vi "_Remote Send Turbo Command.vi"(4 "error in (no error)":errorcluster, 6 "Input Value":i32, 7 "Pump Command":T1) -> (0 "error out":errorcluster, 1 "Data":string, 2 "Raw Reply":string, 3 "Telegram":string)   [LabVIEW 2012]
uses:
  Type/_Pump Parameter.ctl
  Type/_RT Command.ctl
  Type/_RT Serial Command.ctl
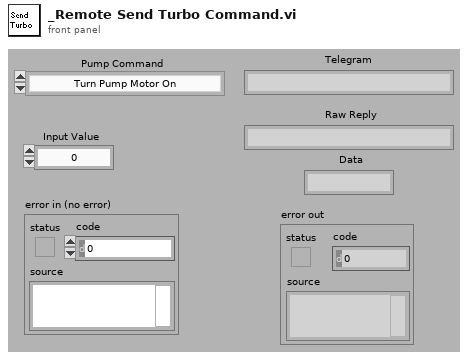
[diagram p1: front panel]
types:
  T1 = typedef "_Pump Parameter.ctl" = enum16{"Turn Pump Motor On", "Turn Pump Motor Off", "Read Pump Oil Deficiency", "Read Rotation Switch Point Attained", "Read Ele. Drive Over Temperature", "Read Pump Over Temperature", "Read Set Rotation Speed Attained", "Read Turbopump Accelerates", "Read Actual Rotation Speed in Hz", "Read Motor Current in A", "Read Operating Hours in h", "Read Motor Voltage in V", "Read Motor Power in W", "Set Rotation Speed Switchpoint in %", "Clear Error", "Read Error Code", "Read Bearing Temperature", "Read Hardware Version", "Read Firmware Version", "Read Operating Hours (Drive)", "Read Rotational Speed (rpm)", "Read Power Stage Temperature", "Read Electronics Temperature", "Read Upper Pump Temperature", "Read Motor Temperature", "Read Error Code History, 1", "Read Error Code History, 2", "Read Error Code History, 3", "Read Error Code History, 4", "Read Error Code History, 5", "Read Error Code History, 6", "Read Error Code History, 7", "Read Error Code History, 8", "Read Error Code History, 9", "Read Error Code History, 10"}
  T2 = typedef "_RT Serial Command.ctl" = cluster{"Port Type":u16, "baud rate (9600)":u32, "data bits (8)":u16, "stop bits (1)":u16, "parity (0:none)":u16, "DoRead":bool, "Command":string}
  T3 = typedef "_RT Command.ctl" = enum16{"Start", "Stop", "Runtime Update", "Get Data", "Get Info", "Get Status", "Get Param", "Get Config", "Get Table", "Read ADC", "Set Oscillator", "Update Config", "Update Table", "Set All Pol", "Set Pol and DC", "Set Max Mass", "Toggle RP", "Toggle EL", "Set PIC", "Initialize Turbo", "Send Turbo Comm", "Close Turbo", "P1", "P2", "P3", "Send Serial", "Set LC Out", "Get LC In", "Read VAC", "Test Table", "Toggle Power", "Get Startup", "Set Startup", "Get ADC Table", "Set ADC Table", "Get Brief Status", "Get Detail Status", "Auxiliary Update", "Set CC Logics", "Set CC Input Logics", "Ignore Error"}
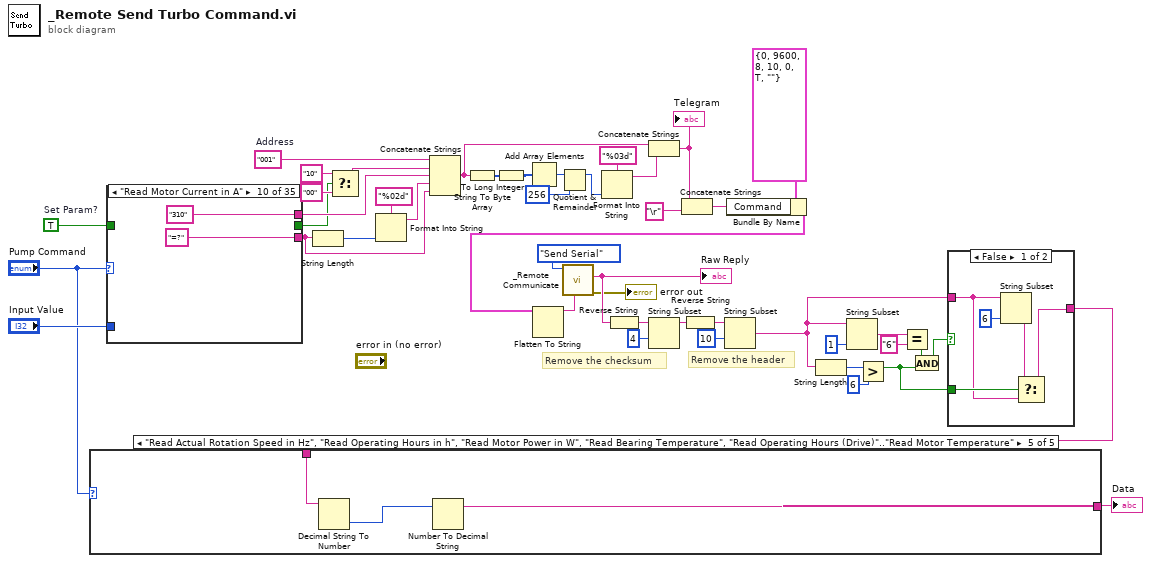
[diagram p0: block diagram]
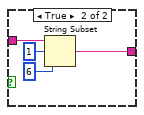
[diagram p2: hidden frame]
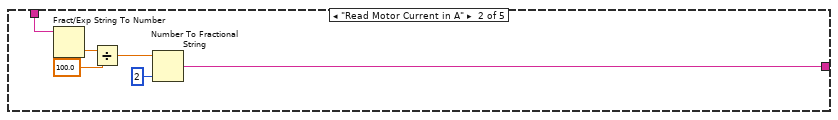
[diagram p4: hidden frame]
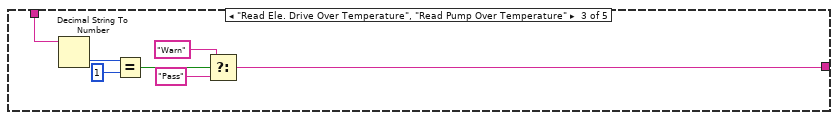
[diagram p5: hidden frame]
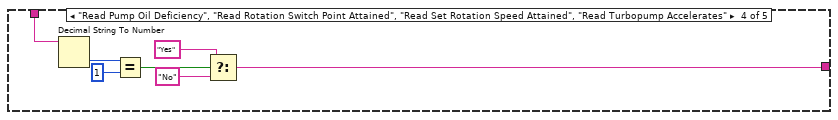
[diagram p6: hidden frame]
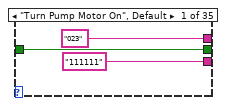
[diagram p7: hidden frame]
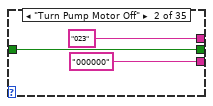
[diagram p8: hidden frame]
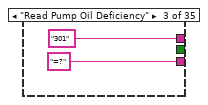
[diagram p9: hidden frame]
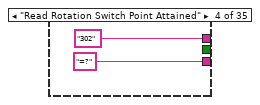
[diagram p10: hidden frame]
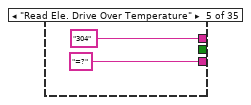
[diagram p11: hidden frame]
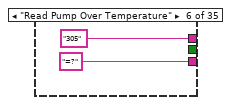
[diagram p12: hidden frame]
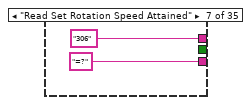
[diagram p13: hidden frame]
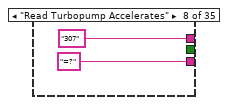
[diagram p14: hidden frame]
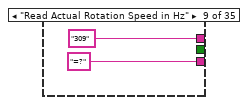
[diagram p15: hidden frame]
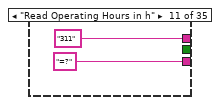
[diagram p16: hidden frame]
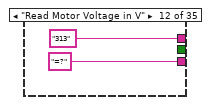
[diagram p17: hidden frame]
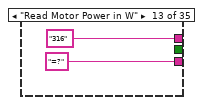
[diagram p18: hidden frame]
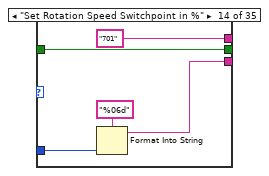
[diagram p19: hidden frame]
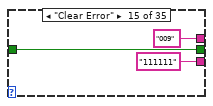
[diagram p20: hidden frame]
diagram:
  w40 = "001"  # Address
  w44 = TRUE  # Set Param?
  # "Remove the header"
  # "Remove the checksum"
  n1 = case shown="\"Read Motor Current in A\"" "Pump Command" {
    tunnel: w44 -> [w49 w50 _ _ _ _ _ _ _ _ _ _ _ w78 w81 _ _ _ _ _ _ _ _ _ _ _ _ _ _ _ _ _ _ _ _]
    tunnel: [w49 w50 _ _ _ _ _ _ _ _ _ _ _ w78 w81 _ _ _ _ _ _ _ _ _ _ _ _ _ _ _ _ _ _ _ _] -> w34
    tunnel: ["023" "023" "301" "302" "304" "305" "306" "307" "309" "310" "311" "313" "316" "701" "009" "303" "342" "354" "312" "314" "398" "324" "326" "330" "346" "360" "361" "362" "363" "364" "365" "366" "367" "368" "369"] -> w35
    tunnel: ["111111" "000000" "=?" "=?" "=?" "=?" "=?" "=?" "=?" "=?" "=?" "=?" "=?" w75 "111111" "=?" "=?" "=?" "=?" "=?" "=?" "=?" "=?" "=?" "=?" "=?" "=?" "=?" "=?" "=?" "=?" "=?" "=?" "=?" "=?"] -> w33
    tunnel: "Input Value" -> [_ _ _ _ _ _ _ _ _ _ _ _ _ w77 _ _ _ _ _ _ _ _ _ _ _ _ _ _ _ _ _ _ _ _ _]
    frame "Turn Pump Motor On", Default {
    }
    frame "Turn Pump Motor Off" {
    }
    frame "Read Pump Oil Deficiency" {
    }
    frame "Read Rotation Switch Point Attained" {
    }
    frame "Read Ele. Drive Over Temperature" {
    }
    frame "Read Pump Over Temperature" {
    }
    frame "Read Set Rotation Speed Attained" {
    }
    frame "Read Turbopump Accelerates" {
    }
    frame "Read Actual Rotation Speed in Hz" {
    }
    frame "Read Motor Current in A" {
    }
    frame "Read Operating Hours in h" {
    }
    frame "Read Motor Voltage in V" {
    }
    frame "Read Motor Power in W" {
    }
    frame "Set Rotation Speed Switchpoint in %" {
      n2 = Format Into String(format string="%06d", w77) -> (resulting string=w75:string)  [unwired: 2 in, 1 out]
    }
    frame "Clear Error" {
    }
    frame "Read Error Code" {
    }
    frame "Read Bearing Temperature" {
    }
    frame "Read Hardware Version" {
    }
    frame "Read Firmware Version" {
    }
    frame "Read Operating Hours (Drive)" {
    }
    frame "Read Rotational Speed (rpm)" {
    }
    frame "Read Power Stage Temperature" {
    }
    frame "Read Electronics Temperature" {
    }
    frame "Read Upper Pump Temperature" {
    }
    frame "Read Motor Temperature" {
    }
    frame "Read Error Code History, 1" {
    }
    frame "Read Error Code History, 2" {
    }
    frame "Read Error Code History, 3" {
    }
    frame "Read Error Code History, 4" {
    }
    frame "Read Error Code History, 5" {
    }
    frame "Read Error Code History, 6" {
    }
    frame "Read Error Code History, 7" {
    }
    frame "Read Error Code History, 8" {
    }
    frame "Read Error Code History, 9" {
    }
    frame "Read Error Code History, 10" {
    }
  }
  n3 = String Length(string=w33) -> (length=w37:i32)
  n4 = Select(t="10", s=w34, f="00") -> (s? t:f=w39:string)
  n5 = Format Into String(format string="%02d", w37) -> (resulting string=w36:string)  [unwired: 2 in, 1 out]
  n6 = Concatenate Strings(w40, w39, w35, w36, w33) -> (w25:string)
  n7 = String To Byte Array(string=w25) -> (unsigned byte array=w26:u8[])
  n8 = To Long Integer(number=w26) -> (32bit integer=w30:i32[])
  n9 = Add Array Elements(numeric array=w30) -> (sum=w32:i32)
  n10 = Quotient & Remainder(x=w32, y=256) -> (x-y*floor(x/y)=w28:i32)  [unwired: 1 out]
  n11 = Format Into String(format string="%03d", w28) -> (resulting string=w27:string)  [unwired: 2 in, 1 out]
  n12 = Concatenate Strings(w25, w27) -> (w24:string)
  "Telegram" <- w24
  n13 = Concatenate Strings(w24, "\r" ("string")) -> (w21:string)
  n14 = Bundle By Name(cluster=T2 {"Port Type"=0, "baud rate (9600)"=9600, "data bits (8)"=8, "stop bits (1)"=10, "parity (0:none)"=0, "DoRead"=TRUE, "Command"=""} ("Serial Command"), "Command"=w21) -> (w20:T2)
  n15 = Flatten To String(anything=w20) -> (data string=w46:string)  [unwired: 1 in, 4 out]
  n16 = call "_Remote Communicate.vi"("String"=w46, "Command"=_RT_Command."Send Serial") -> ("error out"=→"error out":errorcluster, "Info"=w14:string)  [unwired: 4 in, 2 out]
  "Raw Reply" <- w14
  n17 = Reverse String(1:w14) -> (0:w19:string)
  n18 = String Subset(string=w19, offset (0)=4) -> (substring=w15:string)  [unwired: 1 out]
  n19 = Reverse String(1:w15) -> (0:w16:string)
  n20 = String Subset(string=w16, offset (0)=10) -> (substring=w8:string)  [unwired: 1 out]
  n21 = String Length(string=w8) -> (length=w7:i32)
  n22 = String Subset(string=w8, length (rest)=1 ("length (rest)")) -> (substring=w9:string)  [unwired: 1 out]
  n23 = Greater?(x=w7, y=6) -> (0:w3:bool)
  n24 = Equal?(x=w9, y="6") -> (x = y?=w5:bool)
  n25 = And(x=w5, y=w3) -> (x .and. y?=w4:bool)
  n26 = case shown="False" w4 {
    tunnel: w8 -> [w124 w131]
    tunnel: [w123 w128] -> w2
    tunnel: w3 -> [w127 _]
    frame False {
      n27 = String Subset(string=w124, length (rest)=6 ("length (rest)")) -> (substring=w125:string)  [unwired: 1 out]
      n28 = Select(t=w125, s=w127, f=w124) -> (s? t:f=w123:string)
    }
    frame True {
      n29 = String Subset(string=w131, offset (0)=1, length (rest)=6 ("length (rest)")) -> (substring=w128:string)
    }
  }
  n30 = case shown="\"Read Actual Rotation Speed in Hz\", \"Read Operating Hours in h\", \"Read Motor Power in W\", \"Read Bearing Temperature\", \"Read Operating Hours (Drive)\"..\"Read Motor Temperature\"" "Pump Command" {
    tunnel: w2 -> [w132 w138 w145 w152 w155]
    tunnel: [w132 w133 w139 w146 w153] -> w12
    frame "Turn Pump Motor On", Default {
    }
    frame "Read Motor Current in A" {
      n31 = Fract/Exp String To Number(string=w138) -> (number=w137:dbl)  [unwired: 4 out]
      n32 = Divide(x=w137, y=100.0) -> (x/y=w135:dbl)
      n33 = Number To Fractional String(number=w135, precision (6)=i16 2) -> (F-format string=w133:string)  [unwired: 2 out]
    }
    frame "Read Ele. Drive Over Temperature", "Read Pump Over Temperature" {
      n34 = Decimal String To Number(string=w145) -> (number=w144:i32)  [unwired: 3 out]
      n35 = Equal?(x=w144, y=1) -> (x = y?=w142:bool)
      n36 = Select(t="Warn", s=w142, f="Pass") -> (s? t:f=w139:string)
    }
    frame "Read Pump Oil Deficiency", "Read Rotation Switch Point Attained", "Read Set Rotation Speed Attained", "Read Turbopump Accelerates" {
      n37 = Decimal String To Number(string=w152) -> (number=w151:i32)  [unwired: 3 out]
      n38 = Equal?(x=w151, y=1) -> (x = y?=w149:bool)
      n39 = Select(t="Yes", s=w149, f="No") -> (s? t:f=w146:string)
    }
    frame "Read Actual Rotation Speed in Hz", "Read Operating Hours in h", "Read Motor Power in W", "Read Bearing Temperature", "Read Operating Hours (Drive)".."Read Motor Temperature" {
      n40 = Decimal String To Number(string=w155) -> (number=w154:i32)  [unwired: 3 out]
      n41 = Number To Decimal String(number=w154) -> (decimal integer string=w153:string)  [unwired: 1 out]
    }
  }
  "Data" <- w12
